vi "Trav_Space_Edits.vi"(1 "New":T1 {"Min" format="%#.1f"; "Max" format="%#.1f"}, 2 "Original":T1 {"Min" format="%#.1f"; "Max" format="%#.1f"}, 3 "Row Name":string) -> (0 "Changes":string)   [LabVIEW 2011]
uses:
  Box_size.ctl
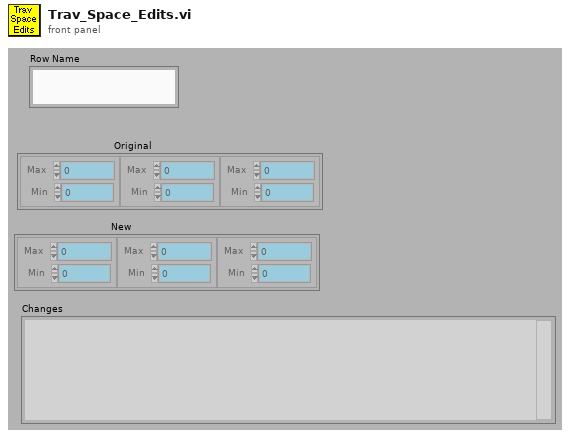
[diagram p1: front panel]
types:
  T1 = typedef "Box_size.ctl" = cluster{"Max":dbl, "Min":dbl}[]
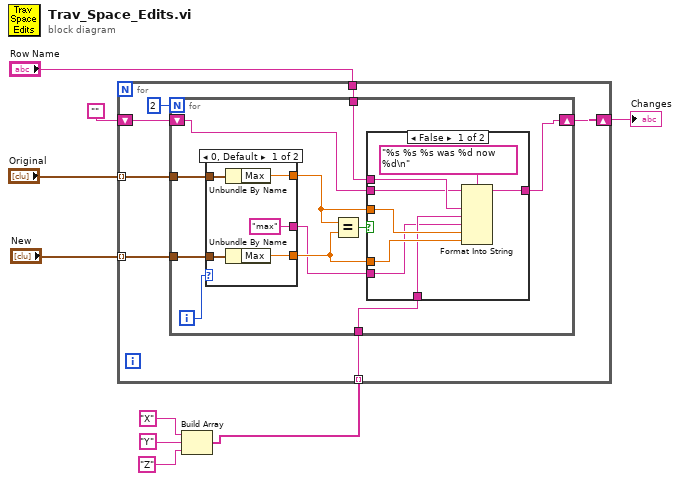
[diagram p0: block diagram]
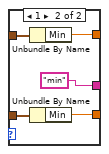
[diagram p2: hidden frame]
diagram:
  n1 = Build Array("X", "Y", "Z") -> (w5:string[])
  n2 = for {
    tunnel: "New" -> [w16] mode=indexing
    tunnel: "Original" -> [w15] mode=indexing
    tunnel: w5 -> [w14] mode=indexing
    tunnel: "Row Name" -> [w13]
    shift-right: [w10] -> w8
    shift-left: "" -> [w11]
    n3 = for {
      N: 2 -> [_]
      tunnel: w16 -> [w27]
      tunnel: w15 -> [w26]
      tunnel: w14 -> [w22]
      tunnel: w13 -> [w21]
      shift-right: [w17] -> w10
      shift-left: w11 -> [w18]
      i -> [w19]
      n4 = case shown="0, Default" w19 {
        tunnel: w27 -> [w32 w37]
        tunnel: w26 -> [w31 w36]
        tunnel: [w30 w35] -> w24
        tunnel: [w29 w34] -> w23
        tunnel: ["max" "min"] -> w20
        frame 0, Default {
          n5 = Unbundle By Name(w31) -> ("Max"=w30:dbl)
          n6 = Unbundle By Name(w32) -> ("Max"=w29:dbl)
        }
        frame 1 {
          n7 = Unbundle By Name(w36) -> ("Min"=w35:dbl)
          n8 = Unbundle By Name(w37) -> ("Min"=w34:dbl)
        }
      }
      n9 = Equal?(x=w24, y=w23) -> (x = y?=w25:bool)
      n10 = case shown="False" w25 {
        tunnel: w24 -> [w45 _]
        tunnel: w23 -> [w44 _]
        tunnel: w22 -> [w41 _]
        tunnel: w21 -> [w42 _]
        tunnel: w20 -> [w40 _]
        tunnel: w18 -> [w39 w46]
        tunnel: [w38 w46] -> w17
        frame False {
          n11 = Format Into String(format string="%s %s %s was %d now  %d\n", initial string=w39, w42, w41, w40, w45, w44) -> (resulting string=w38:string)  [unwired: 1 in, 1 out]
        }
        frame True {
        }
      }
    }
  }
  "Changes" <- w8
